vi "Save Test Information to DB.vi"(8 "error in (no error)":errorcluster, 11 "Cluster":T1) -> (0 "error out":errorcluster)   [LabVIEW 2017]
uses:
  Controls/Testscreen_Input cluster.ctl
  <vilib>/addons/database/Connection.llb/Conn ObjectReference.ctl
  <vilib>/addons/database/NI_Database_API.lvlib
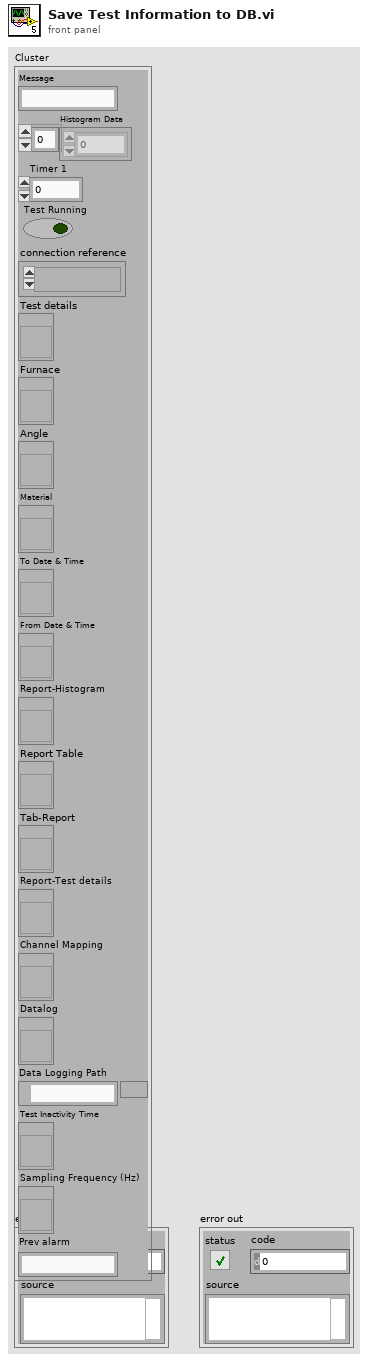
[diagram p1: front panel]
types:
  T1 = typedef "Testscreen_Input cluster.ctl" = cluster{"Message":string, "Histogram Data":i32[], "Timer 1":u32, "Test Running":bool, "connection reference":T2, "Test details":refnum<vi>, "Furnace":refnum<vi>, "Angle":refnum<vi>, "Material":refnum<vi>, "To Date & Time":refnum<vi>, "From Date & Time":refnum<vi>, "Report-Histogram":refnum<vi>, "Report Table":refnum<vi>, "Tab-Report":refnum<vi>, "Report-Test details":refnum<vi>, "Channel Mapping":refnum<vi>, "Datalog":refnum<vi>, "Data Logging Path":path, "Test Inactivity Time":refnum<vi>, "Sampling Frequency (Hz)":refnum<vi>, "Prev alarm":string}
  T2 = typedef "NI_Database_API.lvlib/Conn ObjectReference.ctl" = refnum<k1>
  T3 = cluster{"ID":string, "Test Name":string, "Flowrate":string, "Furnace":string, "Material":string, "Angle":string, "Tested By":string}
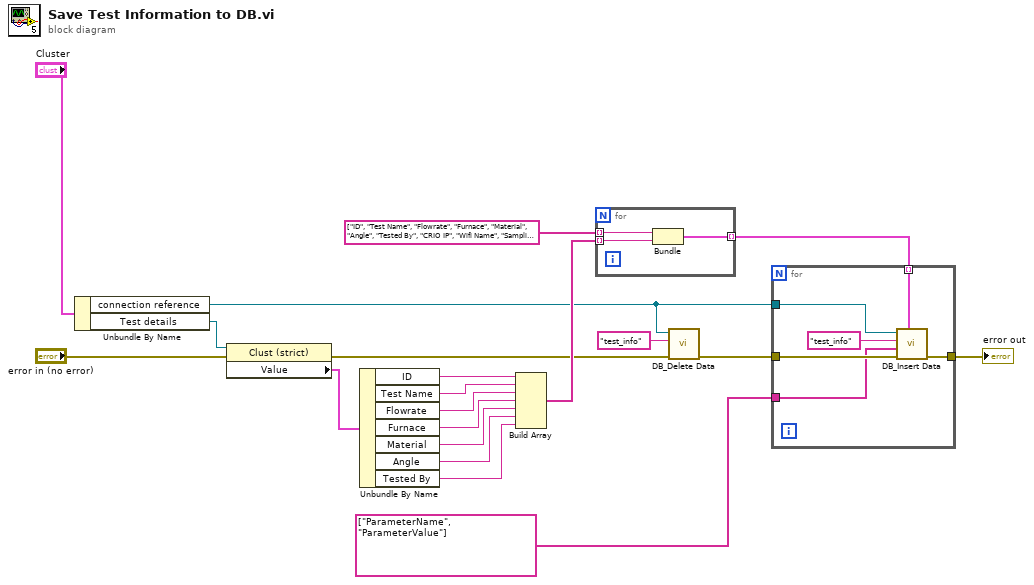
[diagram p0: block diagram]
diagram:
  n1 = Unbundle By Name("Cluster") -> ("connection reference"=w11:T2, "Test details"=w2:refnum<vi>)
  n2 = property class="Clust (strict)"(reference=w2, error in="error in (no error)") -> (error out=w12:errorcluster, "Value"=w19:T3)  [unwired: 1 out]
  n3 = Unbundle By Name(w19) -> ("ID"=w4:string, "Test Name"=w5:string, "Flowrate"=w6:string, "Furnace"=w7:string, "Material"=w8:string, "Angle"=w9:string, "Tested By"=w10:string)
  n4 = Build Array(w4, w5, w6, w7, w8, w9, w10) -> (w16:string[])
  n5 = for {
    tunnel: string[] ["ID", "Test Name", "Flowrate", "Furnace", "Material", "Angle", "Tested By", "CRIO IP", "Wifi Name", "Sampling Frequency", "Test Inactivity Time", "Drive Path"] ("columns") -> [w23] mode=indexing
    tunnel: w16 -> [w22] mode=indexing
    tunnel: [w21] -> w18 mode=indexing
    n6 = Bundle("String"=w23, "Tested By"=w22) -> (w21:cluster{"String":string, "Tested By":string})  [unwired: 1 in]
  }
  n7 = call "DB_Delete Data.vi"("error in (no error)"=w12, "table"="test_info", "connection reference"=w11) -> ("error out"=w13:errorcluster)  [unwired: 8 in]
  n8 = for {
    tunnel: w11 -> [w27]
    tunnel: string[] ["ParameterName", "ParameterValue"] ("table") -> [w25]
    tunnel: w13 -> [w26]
    tunnel: [w29] -> w20
    tunnel: w18 -> [w24] mode=indexing
    n9 = call "DB_Insert Data.vi"("data"=w24, "error in (no error)"=w26, "columns"=w25, "table"="test_info", "connection reference"=w27) -> ("error out"=w29:errorcluster)  [unwired: 6 in]
  }
  "error out" <- w20
